vi "format mapping info.vi"(9 "instance id":string, 10 "channel":refnum<class "TBM channel.lvclass">, 11 "engine configuration in":refnum<class "engine configuration.lvclass">) -> (3 "mapping info":string)   [LabVIEW 2013, in "control module editor.lvclass"]
uses:
  control module editor.lvclass
  <vilib>/NI/Tag Bus Module Framework/channel/TBM channel.lvclass
  <vilib>/NI/Module Execution Interface/Engine Configuration/engine configuration.lvclass
  <vilib>/NI/Tag Bus/tag/tag descriptor.lvclass/tag descriptor.ctl
  <vilib>/NI/Tag Bus/tag/tag descriptor.lvclass
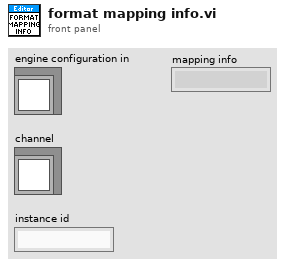
[diagram p1: front panel]
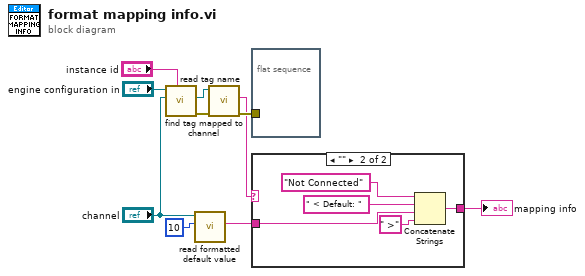
[diagram p0: block diagram]
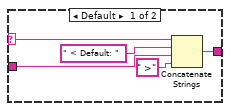
[diagram p2: hidden frame]
diagram:
  n1 = call <vilib>:"find tag mapped to channel.vi"("owner"="instance id", "channel"="channel", "engine configuration in"="engine configuration in") -> ("error out"=w4:errorcluster, "tag"=w2:refnum<class "tag descriptor.lvclass">)  [unwired: 6 in, 1 out]
  n2 = call "read formatted default value.vi"("# of Digits"=10 ("y"), "channel"="channel") -> ("Formatted Default"=w10:string)  [unwired: 8 in, 1 out]
  n3 = call <vilib>:"read tag name.vi"("error in"=w4, "system tag in"=w2) -> ("error out"=w7:errorcluster, "name"=w5:string)  [unwired: 7 in, 1 out]
  n4 = flat-sequence {
    tunnel: w7 -> [_]
    frame #0 {
    }
  }
  n5 = case shown="\"\"" w5 {
    selector: w5 -> [w12 _]
    tunnel: [w11 w17] -> w6
    tunnel: w10 -> [w13 w16]
    frame Default {
      n6 = Concatenate Strings(w12, " < Default: " ("string"), w13, " >" ("string")) -> (w11:string)
    }
    frame "" {
      n7 = Concatenate Strings("Not Connected", " < Default: " ("string"), w16, " >" ("string")) -> (w17:string)
    }
  }
  "mapping info" <- w6
